vi "RichToFlatlogging_service_LogResponse.vi"(5 "OutputClusterType":T1, 11 "InputCluster":T2) -> (3 "OutputCluster":T1)   [LabVIEW 2023, in "logmeasurement_client.lvlib"]
uses:
  logging_service_LogResponse.ctl
  logging_service_LogResponse_Flat.ctl
  logmeasurement_client.lvlib
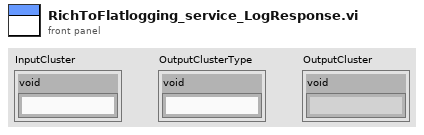
[diagram p1: front panel]
types:
  T1 = typedef "logmeasurement_client.lvlib/logging_service_LogResponse_Flat.ctl" = cluster{"void":string}
  T2 = typedef "logmeasurement_client.lvlib/logging_service_LogResponse.ctl" = cluster{"void":string}
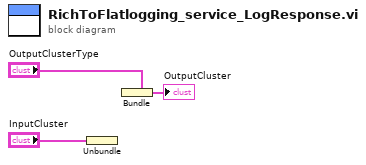
[diagram p0: block diagram]
diagram:
  n1 = Unbundle "Unbundle"("InputCluster") -> ()  [unwired: 1 out]
  n2 = Bundle "Bundle"(cluster="OutputClusterType") -> (→"OutputCluster":T1)  [unwired: 1 in]
